vi "Generate Sine and Cosine.vi"(1 "Amplitude":dbl, 2 "Number of Samples":dbl) -> (0 "Waveform Graph":dbl[][](graph))   [LabVIEW 2021]
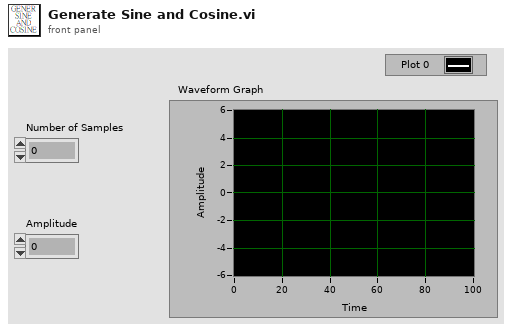
[diagram p1: front panel]
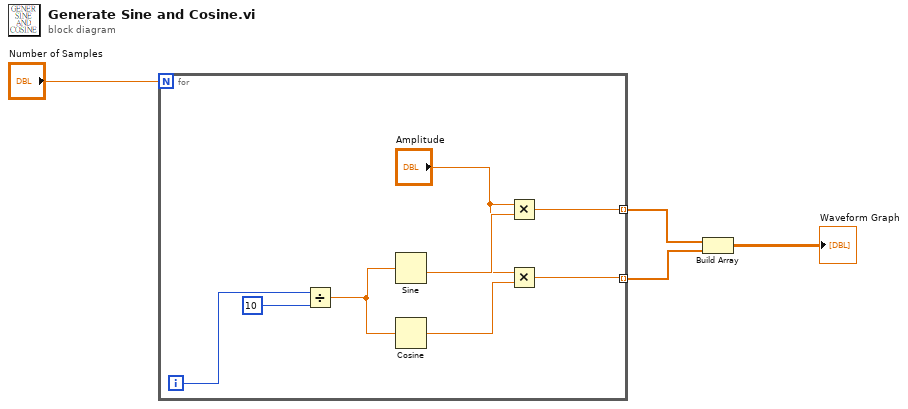
[diagram p0: block diagram]
diagram:
  n1 = for {
    N: "Number of Samples" -> [_]
    tunnel: [w6] -> w2 mode=indexing
    tunnel: [w5] -> w3 mode=indexing
    i -> [w12]
    n2 = Divide(x=w12, y=10) -> (x/y=w11:dbl)
    n3 = Sine(x=w11) -> (sin(x)=w9:dbl)
    n4 = Cosine(x=w11) -> (cos(x)=w8:dbl)
    n5 = Multiply(x="Amplitude", y=w9) -> (x*y=w5:dbl)
    n6 = Multiply(x="Amplitude", y=w8) -> (x*y=w6:dbl)
  }
  n7 = Build Array(w3, w2) -> (→"Waveform Graph":dbl[][])
